vi "temp-conv (SubVI).vi"(9 "Slide 2":dbl(slide) scale=0.0..10.0, 10 "Slide":dbl(slide) scale=0.0..300.0, 11 "Deg  F":dbl) -> (3 "Deg C":dbl)   [LabVIEW 2015]
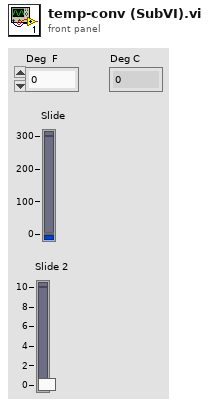
[diagram p1: front panel]
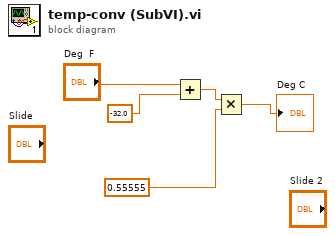
[diagram p0: block diagram]
diagram:
  n1 = Add(x="Deg  F", y=-32.0 ("deg C")) -> (x+y=w2:dbl)
  n2 = Multiply(x=w2, y=0.55555) -> (x*y=→"Deg C":dbl)
